vi "Actor Core.vi"(8 "error in":errorcluster, 11 "Example View in":refnum<class "Example GUI View.lvclass">) -> (0 "error out":errorcluster, 3 "Actor out":refnum<class "Actor.lvclass">)   [LabVIEW 2023, in "Example GUI View.lvlib" / "Example GUI View.lvclass"]
doc: "(<B>Filename</B>: Actor Framework.lvlib:Actor.lvclass:Actor Core.vi)\n\nReceives messages to the actor, reacts to them, and initiates any error handling that may shut the actor down.\n\nDescendant classes may override this VI to append parallel tasks for the actor to complete while it handles messages. Overrides use the Call Parent Method node."
uses:
  Example GUI View.lvclass
  <vilib>/ActorFramework/Actor/Actor.lvclass
  Example GUI View.lvclass/Example GUI View.ctl
  <vilib>/ActorFramework/Actor/Actor.lvclass/Actor.ctl
  <vilib>/ActorFramework/Message Enqueuer/Message Enqueuer.lvclass/Message Enqueuer.ctl
  View/View.lvclass/View.ctl
  Example Events/Boolean Event.lvclass
  View/properties/Read Name.vi
  <vilib>/ActorFramework/Message Enqueuer/Init from Existing Queue.vi
  <vilib>/ActorFramework/Message Enqueuer/Message Enqueuer.lvclass
  GUI Views/GUI View/GUI View.lvclass
  View Messages/Generate and Broadcast Event Msg/Generate and Broadcast Event Msg.lvclass
panel:
  out "View Name":string
  in  "Boolean":bool
  out "Time":string
  out "Waveform Graph":dbl[](graph)
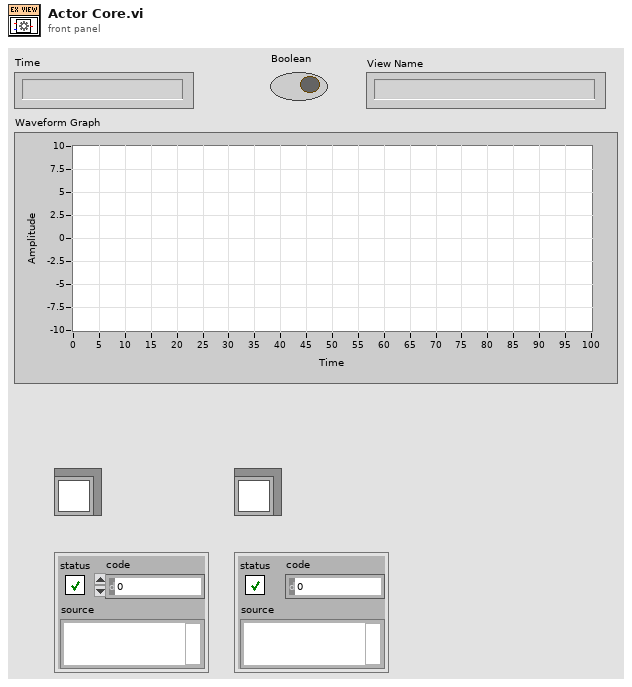
[diagram p1: front panel]
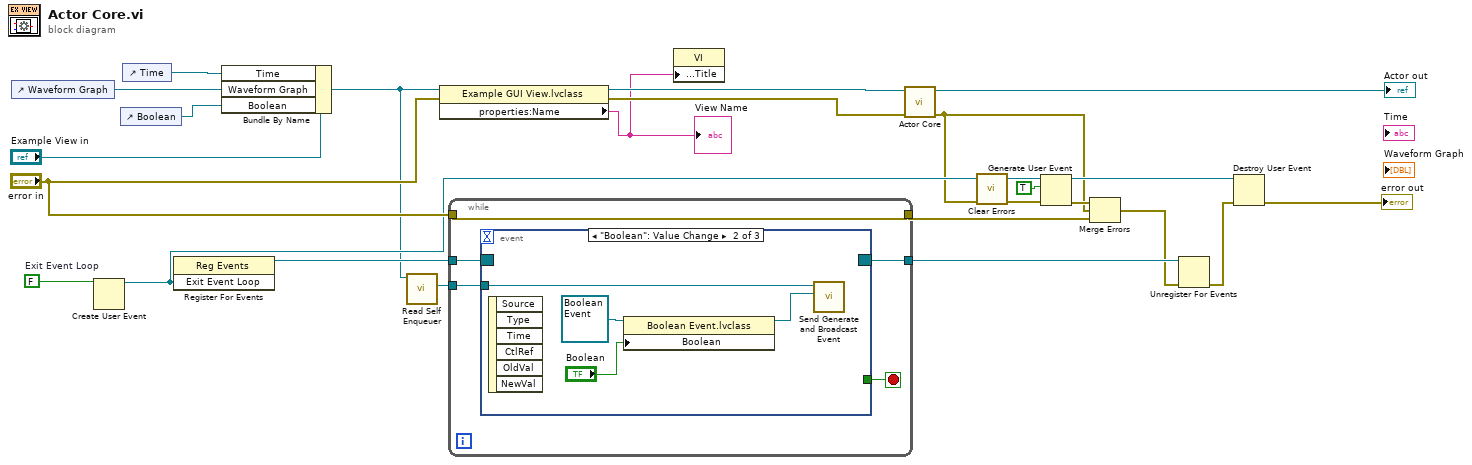
[diagram p0: block diagram]
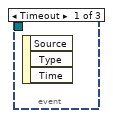
[diagram p2: hidden frame]
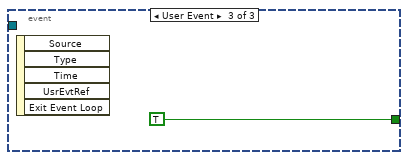
[diagram p3: hidden frame]
diagram:
  w17 = FALSE  # Exit Event Loop
  n1 = control-ref of="Waveform Graph"() -> (w21:refnum<vi>)
  n2 = Create User Event(user event datatype=w17) -> (user event=w14:refnum<user-event>)  [unwired: 1 in, 1 out]
  n3 = control-ref of="Boolean"() -> (w20:refnum<vi>)
  n4 = control-ref of="Time"() -> (w22:refnum<vi>)
  n5 = register-events(w14) -> (reference out=w16:refnum<event-registration>)  [unwired: 2 in, 1 out]
  n6 = Bundle By Name(cluster="Example View in", "Time"=w22, "Waveform Graph"=w21, "Boolean"=w20) -> (w9:refnum<class "Example GUI View.lvclass">)
  n7 = call <vilib>:"Read Self Enqueuer.vi"("Actor"=w9) -> ("Self Enqueuer"=w18:refnum<class "Message Enqueuer.lvclass">)  [unwired: 10 in]
  n8 = property class="Example GUI View.lvclass"(reference=w9, error in="error in") -> (reference out=w3:refnum<class "Example GUI View.lvclass">, error out=w2:errorcluster, "properties:Name"=w1:string)
  "View Name" <- w1
  n9 = while {
    tunnel: w18 -> [w29]
    tunnel: w16 -> [w28]
    tunnel: "error in" -> [w27]
    tunnel: [w27] -> w8
    tunnel: [w26] -> w12
    stop <- w25 stop-if-true
    n10 = event shown="[1] \"Boolean\": Value Change" {
      selector: w28 -> [_ _ _]
      dyn-events: [_ _ _] -> w26
      timeout: _ -> [_ _ _]
      tunnel: w29 -> [_ w33 _]
      tunnel: [_ _ TRUE] -> w25
      event Timeout {
        n11 = event-data() -> ()  [unwired: 1 in, 3 out]
      }
      event "Boolean": Value Change {
        n12 = event-data() -> ()  [unwired: 1 in, 6 out]
        n13 = property class="Boolean Event.lvclass"(reference=refnum<class "Boolean Event.lvclass"> refnum ("Example Source.lvlib:Boolean Event.lvclass"), "Boolean"="Boolean") -> (reference out=w30:refnum<class "Boolean Event.lvclass">)  [unwired: 1 in, 1 out]
        n14 = call "Send Generate and Broadcast Event.vi"("Event Data"=w30, "Message Enqueuer in"=w33) -> ()  [unwired: 8 in, 2 out]
      }
      event User Event {
        n15 = event-data() -> ()  [unwired: 1 in, 5 out]
      }
    }
  }
  n16 = property class="VI"("Front Panel.Title"=w1) -> ()  [unwired: 2 in, 2 out]
  n17 = call-parent "Actor Core.vi"("error in"=w2, "GUI View in"=w3) -> ("error out"=w5:errorcluster, "Actor out"=→"Actor out":refnum<class "Actor.lvclass">)  [unwired: 8 in]
  n18 = call <vilib>:"Clear Errors.vi"("error in (no error)"=w5) -> ("error out"=w4:errorcluster)  [unwired: 5 in, 1 out]
  n19 = Generate User Event(user event=w14, event data cluster=TRUE ("event data"), error in=w4) -> (user event out=w13:refnum<user-event>, error out=w15:errorcluster)  [unwired: 1 in]
  n20 = Merge Errors(w15, w5, w8) -> (w6:errorcluster)
  n21 = Unregister For Events(event registration refnum=w12, error in=w6) -> (error out=w11:errorcluster)
  n22 = Destroy User Event(user event=w13, error in=w11) -> (error out=→"error out":errorcluster)
